vi "read magnetometer values.vi"() -> ()   [LabVIEW 2019]
uses:
  <vilib>/rvi/Emulation/niFpgaGetClockAttributes.vi
  <vilib>/rvi/Emulation/niFpgaSctlEmulationGetInTimedLoop.vi
  <vilib>/rvi/Emulation/niFpgaEmulationReportErrorSimple.vi
  <vilib>/rvi/Emulation/niFpgaCriticalErrorInLSC.vi
panel:
  out "Z":i16
  out "X":i16
  out "Y":i16
  in  "[ESC]":bool
  out "Waveform Chart":cluster{i16, i16, i16}(graph)
  out "ACK3":bool
  out "SDA3":bool
  in  "add + read bite":u8 format="%x"
  out "adress + READ booleans":bool[](array[boolean])
  out "ACK2":bool
  out "SDA2":bool
  in  "register":u8 format="%x"
  out "register adress":bool[](array[boolean])
  out "SDA1":bool
  out "ACK1":bool
  in  "adresse + Write":u8 format="%x"
  out "Adresse + command byte":bool[](array[boolean])
  # "read magnetometer values"
  # "3D"
  # "3C"
  # "E8"
  # "0x68 ,  we have to set the MSB to 1, making the subaddress 0xE8"
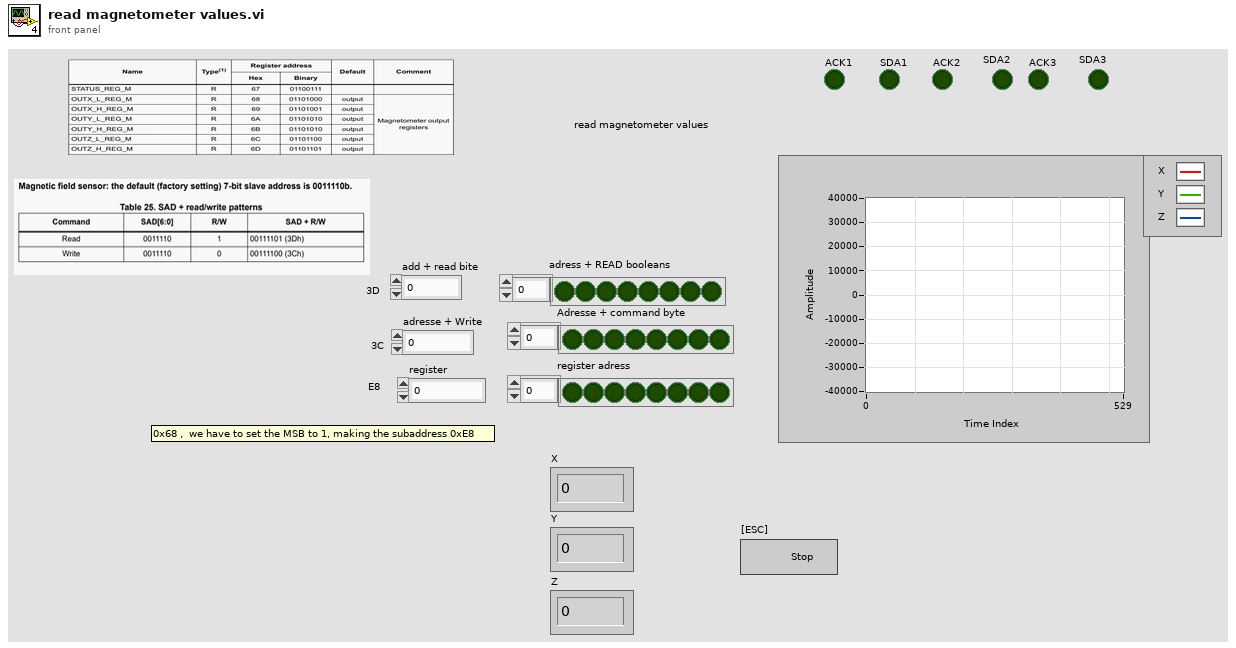
[diagram p1: front panel]
types:
  T1 = cluster{"Raw X axis ":i16, "Raw Y axis ":i16, "Raw Z axis ":i16}
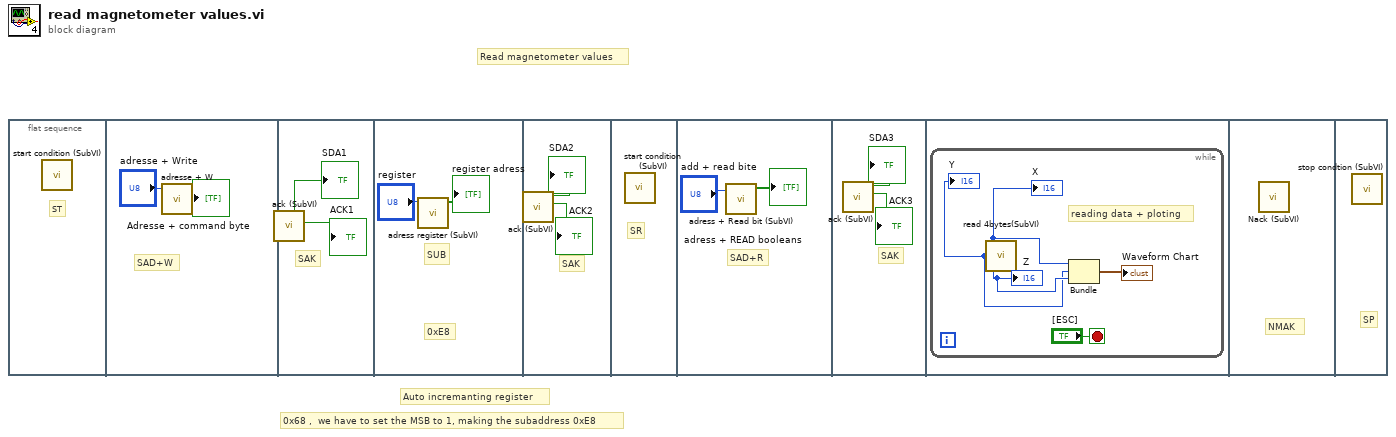
[diagram p0: block diagram]
diagram:
  # "0x68 ,  we have to set the MSB to 1, making the subaddress 0xE8"
  # "Read magnetometer values"
  # "Auto incremanting register"
  n1 = flat-sequence {
    frame #0 {
      # "ST"
      n2 = call "start condition (SubVI).vi"() -> ()  [unwired: 12 in]
    }
    frame #1 {
      # "SAD+W"
      n3 = call "adresse + W.vi"("adresse + Write"="adresse + Write") -> ("Adresse + command byte"=→"Adresse + command byte":bool[])  [unwired: 10 in]
    }
    frame #2 {
      # "SAK"
      n4 = call "ack (SubVI).vi"() -> ("ACK"=→"ACK1":bool, "SDA"=→"SDA1":bool)  [unwired: 10 in]
    }
    frame #3 {
      # "0xE8"
      # "SUB"
      n5 = call "adress register (SubVI).vi"("register"="register") -> ("register adress"=→"register adress":bool[])  [unwired: 10 in]
    }
    frame #4 {
      # "SAK"
      n6 = call "ack (SubVI).vi"() -> ("ACK"=→"ACK2":bool, "SDA"=→"SDA2":bool)  [unwired: 10 in]
    }
    frame #5 {
      # "SR"
      n7 = call "start condition (SubVI).vi"() -> ()  [unwired: 12 in]
    }
    frame #6 {
      # "SAD+R"
      n8 = call "adress + Read bit (SubVI).vi"("add + read bite"="add + read bite") -> ("adress + R booleans"=→"adress + READ booleans":bool[])  [unwired: 10 in]
    }
    frame #7 {
      # "SAK"
      n9 = call "ack (SubVI).vi"() -> ("ACK"=→"ACK3":bool, "SDA"=→"SDA3":bool)  [unwired: 10 in]
    }
    frame #8 {
      n10 = while {
        stop <- "[ESC]" stop-if-true
        # "reading data + ploting"
        n11 = call "read 4bytes(SubVI).vi"() -> ("Raw Z axis"=w16:i16, "Raw Y axis"=w15:i16, "Raw X axis"=w17:i16)  [unwired: 1 in]
        "Z" <- w16
        "X" <- w17
        "Y" <- w15
        n12 = Bundle("Raw X axis"=w17, "Raw Y axis"=w15, "Raw Z axis"=w16) -> (→"Waveform Chart":T1)  [unwired: 1 in]
      }
    }
    frame #9 {
      # "NMAK"
      n13 = call "Nack (SubVI).vi"() -> ()  [unwired: 12 in]
    }
    frame #10 {
      # "SP"
      n14 = call "stop condtion (SubVI).vi"() -> ()  [unwired: 12 in]
    }
  }
